vi "Radar_2channel_DAQ.vi"() -> ()   [LabVIEW 2014]
doc: "Personal Daq 54 example.\nTriggering is immediate and readings are returned 1 scan at a time as available.\nBe sure to use the Acquisition Stop control for proper shutdown."
uses:
  <vilib>/Utility/error.llb/DialogType.ctl
  <vilib>/DAQmx/read.llb/DAQmx Read (Analog 1D DBL NChan 1Samp).vi
  <vilib>/Analysis/2dsp.llb/Complex FFT.vi
  <vilib>/DAQmx/create/channels.llb/DAQmx Create Channel (AI-Voltage-Basic).vi
  <vilib>/DAQmx/configure/timing.llb/DAQmx Timing (Sample Clock).vi
  <vilib>/DAQmx/miscellaneous.llb/DAQmx Fill In Error Info.vi
  <vilib>/measure/madcrms.llb/Basic Averaged DC-RMS for 1 Chan.vi
  <vilib>/Analysis/NI_AALPro.lvlib
  <vilib>/measure/NI_MAPro.lvlib
panel:
  in  "Q Channel":i32=1
  in  "I Channel":i32
  in  "Terminal Config":i32(ring)=10083 items=["Default"=-1, "RSE"=10083, "NRSE"=10078, "Differential"=10106, "Pseudodifferential"=12529]
  out "Filename Out":path
  in  "Physical Channels":string(combo)="Dev1/ai0:7"
  out "I/Q Signal":dynamicdata(graph)
  in  "Save Data":bool
  in  "stop":bool
  in  "Max Voltage":dbl=5.0 caption="Maximum Value"
  in  "Min Voltage":dbl caption="Minimum Value"
  in  "Rate":dbl=20.0 caption="Sample Rate (Hz)" format="%0.2f"
  in  "Samples per Channel":i32=1
  out "Spectrum":waveform(dbl)(graph)
  in  "Data Length":i32=256
  # "Interferometry Radar Processing with NI USB-DAQ"
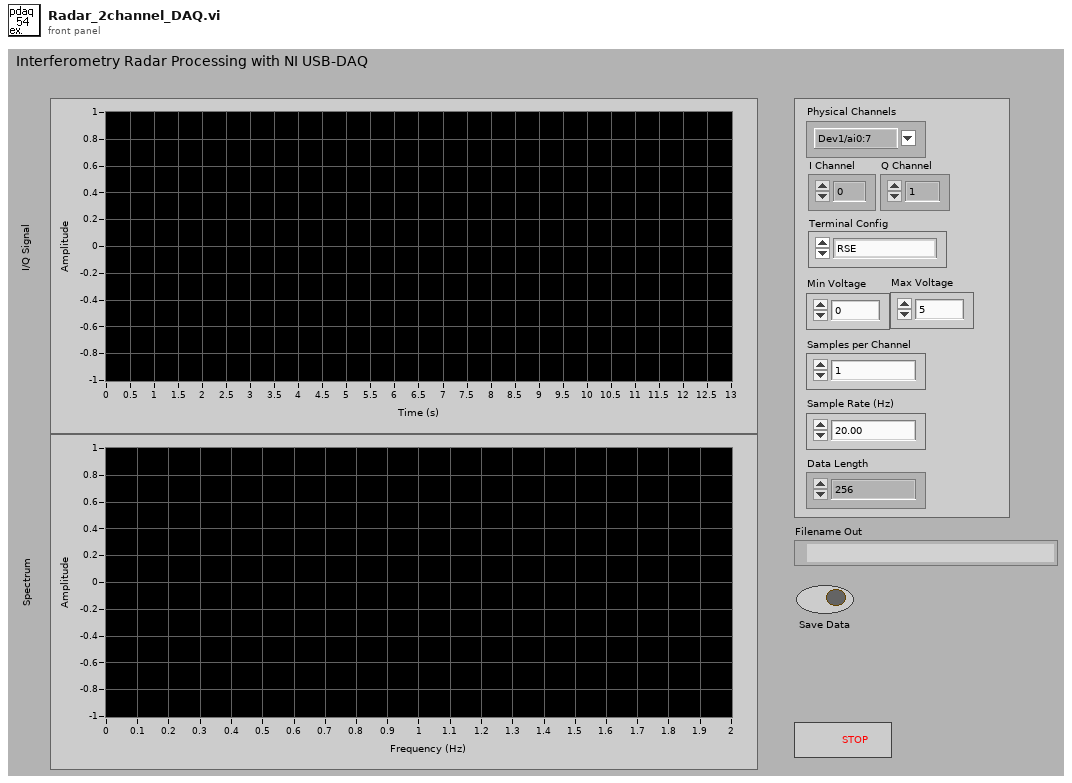
[diagram p1: front panel]
types:
  T1 = typedef "DialogType.ctl" = u16
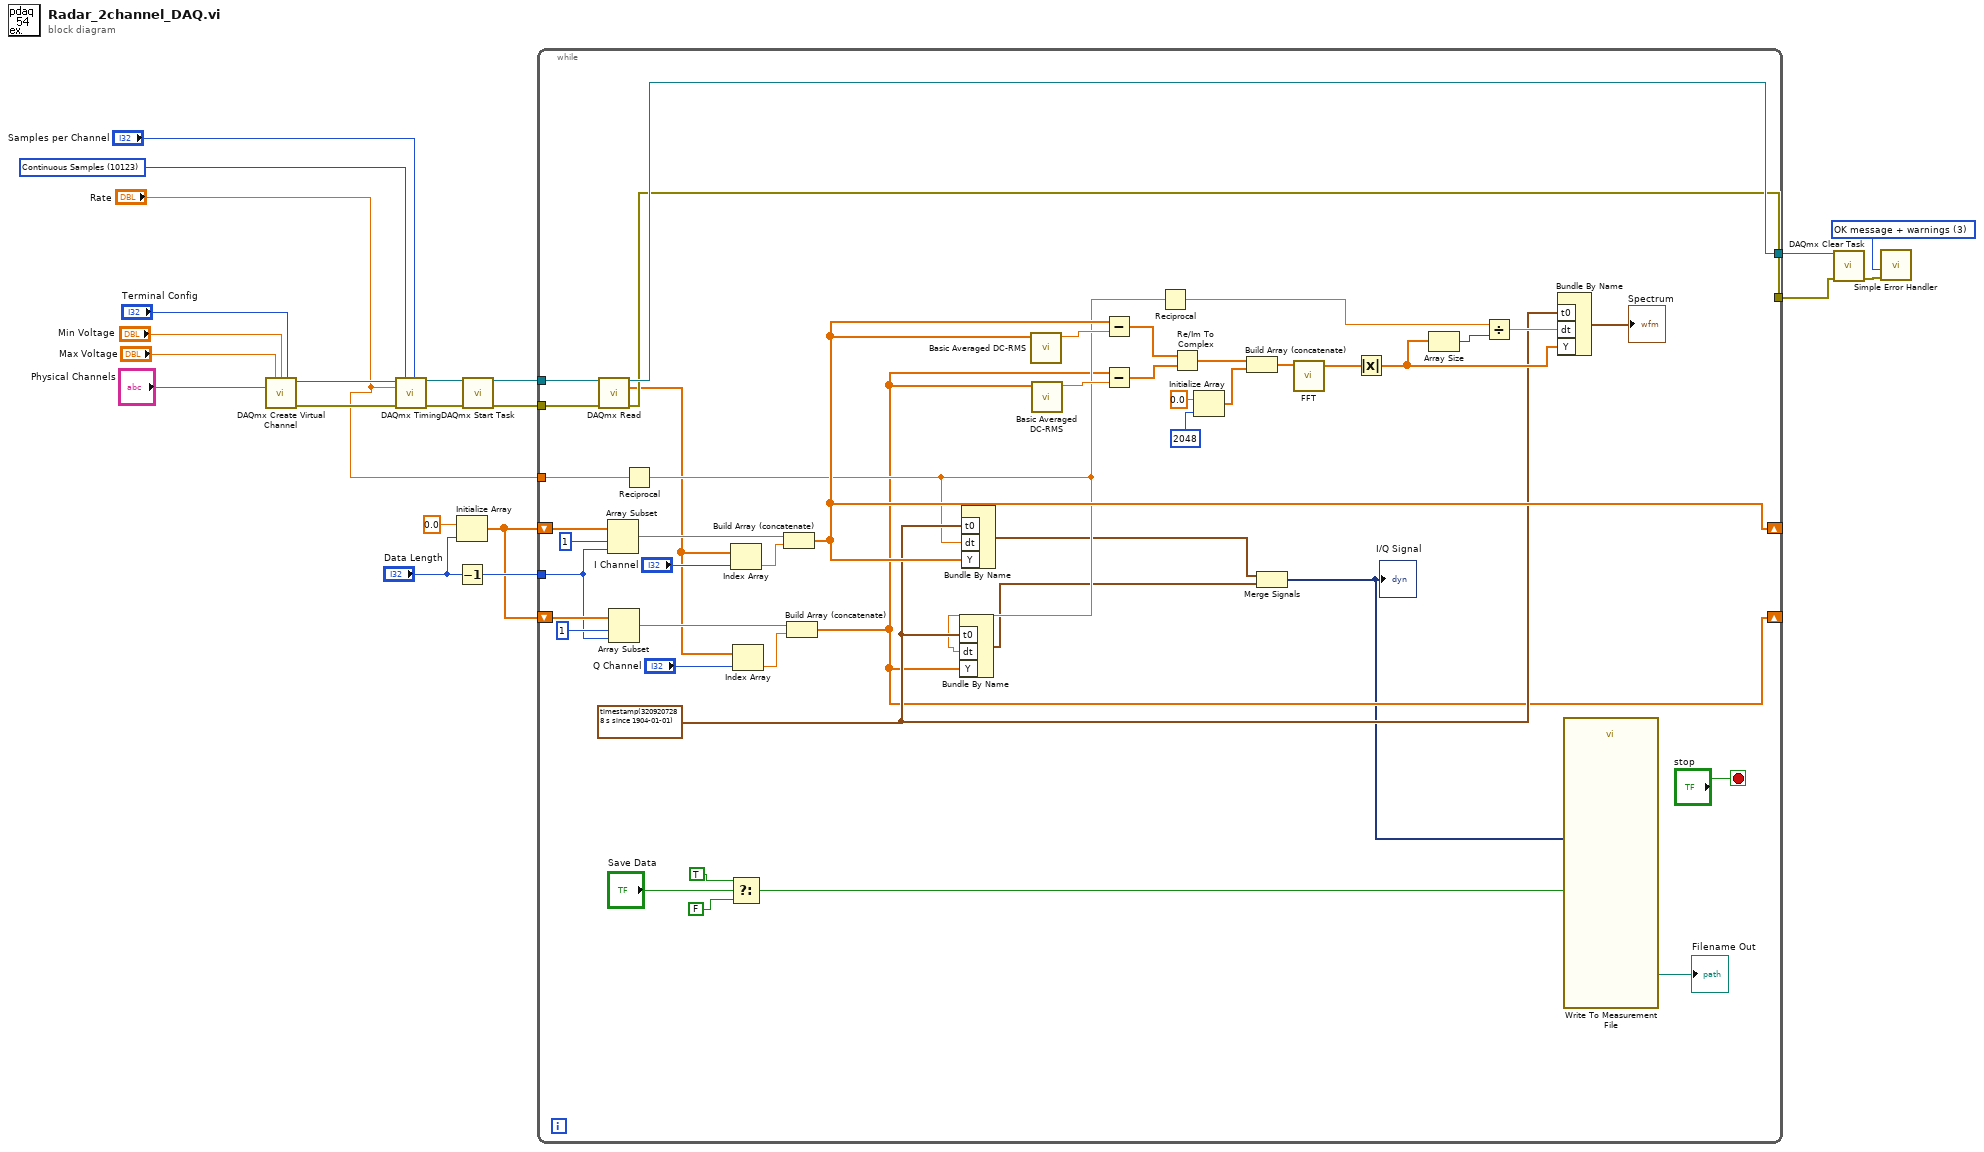
[diagram p0: block diagram]
diagram:
  w7 = T1 3 items=["no dialog", "OK message", "continue or stop message", "OK message + warnings", "continue/stop + warnings"] ("type of dialog (OK msg:1)")
  w14 = 10123 items=["Finite Samples"=10178, "Continuous Samples"=10123] ("sample mode")
  n1 = call-poly <vilib>:"DAQmx Create Virtual Channel.vi"("maximum value"="Max Voltage", "minimum value"="Min Voltage", "input terminal configuration"="Terminal Config", "physical channels"="Physical Channels") -> ("task out"=w15:refnum<k21>, "error out"=w17:errorcluster)  [unwired: 5 in, 5 out]
  n2 = call-poly <vilib>:"DAQmx Timing.vi"("task/channels in"=w15, "sample mode"=w14, "samples per channel"="Samples per Channel", "rate"="Rate", "error in"=w17) -> ("task out"=w13:refnum<k21>, "error out"=w12:errorcluster)  [unwired: 2 in, 7 out]
  n3 = Initialize Array(0.0 ("element"), "Data Length") -> (w2:dbl[])
  n4 = Decrement(x="Data Length") -> (x-1=w20:i32)
  n5 = call <vilib>:"DAQmx Start Task.vi"("task/channels in"=w13, "error in"=w12) -> ("task out"=w10:refnum<k21>, "error out"=w9:errorcluster)  [unwired: 12 out]
  n6 = while {
    shift-right: [w51] -> _
    shift-left: w2 -> [w65]
    tunnel: w20 -> [w38]
    shift-right: [w25] -> _
    shift-left: w2 -> [w63]
    tunnel: w10 -> [w50]
    tunnel: w9 -> [w49]
    tunnel: "Rate" -> [w48]
    tunnel: [w47] -> w6
    tunnel: [w46] -> w5
    stop <- "stop" stop-if-true
    w36 = timestamp(3209207288.296 s since 1904-01-01) ("t0")
    n7 = call-poly <vilib>:"DAQmx Read.vi"("task/channels in"=w50, "error in"=w49) -> ("task out"=w47:refnum<k21>, "data"=w28:dbl[], "error out"=w46:errorcluster)  [unwired: 11 out]
    n8 = Array Subset(array=w65, index=1, length=w38) -> (w29:dbl[])
    n9 = Array Subset(array=w63, index=1, length=w38) -> (w61:dbl[])
    n10 = Reciprocal(x=w48) -> (1/x=w35:dbl)
    n11 = Index Array(array=w28, index="I Channel") -> (element=w27:dbl)
    n12 = Select(t=TRUE, s="Save Data", f=FALSE) -> (s? t:f=w23:bool)
    n13 = Index Array(array=w28, index="Q Channel") -> (element=w26:dbl)
    n14 = Build Array (concatenate)(w29, w27) -> (w51:dbl[])
    n15 = Build Array (concatenate)(w61, w26) -> (w25:dbl[])
    n16 = Bundle By Name("t0"=w36, "dt"=w35, "Y"=w25) -> (w30:waveform(dbl))  [unwired: 1 out]
    n17 = Bundle By Name("t0"=w36, "dt"=w35, "Y"=w51) -> (w31:waveform(dbl))  [unwired: 1 out]
    n18 = call-poly <vilib>:"Basic Averaged DC-RMS.vi"("signal in"=w51) -> ("DC value"=w56:dbl)  [unwired: 4 in, 6 out]
    n19 = call-poly <vilib>:"Basic Averaged DC-RMS.vi"("signal in"=w25) -> ("DC value"=w57:dbl)  [unwired: 4 in, 6 out]
    n20 = Subtract(x=w51, y=w56) -> (x-y=w44:dbl[])
    n21 = Subtract(x=w25, y=w57) -> (x-y=w43:dbl[])
    n22 = Reciprocal(x=w35) -> (1/x=w41:dbl)
    n23 = Re/Im To Complex(1:w43, 2:w44) -> (0:w58:cdb[])
    n24 = Initialize Array(0.0 ("element"), 2048 ("dimension size")) -> (w37:dbl[])
    n25 = Build Array (concatenate)(w58, w37) -> (w52:cdb[])
    n26 = Merge Signals(w31, w30) -> (w24:dynamicdata)
    "I/Q Signal" <- w24
    n27 = call-poly <vilib>:"FFT.vi"("X"=w52) -> ("FFT {X}"=w55:cdb[])  [unwired: 2 in, 8 out]
    n28 = Absolute Value(x=w55) -> (abs(x)=w39:dbl[])
    n29 = Array Size(array=w39) -> (size(s)=w53:i32)
    n30 = Divide(x=w41, y=w53) -> (x/y=w40:dbl)
    n31 = Bundle By Name("t0"=w36, "dt"=w40, "Y"=w39) -> (→"Spectrum":waveform(dbl))  [unwired: 1 out]
    n32 = call "Write To Measurement File"("Signals"=w24, "Enable"=w23) -> ("Filename Out"=→"Filename Out":path)  [unwired: 15 in, 2 out]
  }
  n33 = call <vilib>:"DAQmx Clear Task.vi"("task in"=w6, "error in"=w5) -> ("error out"=w4:errorcluster)  [unwired: 13 out]
  n34 = call <vilib>:"Simple Error Handler.vi"("type of dialog (OK msg:1)"=w7, "error in (no error)"=w4) -> ()  [unwired: 8 out]
